vi "Shoot_object.vi"(7 "Shoot_states":T1, 8 "error in":errorcluster, 11 "DataIn":variant) -> (0 "error out":errorcluster)   [LabVIEW 2017]
uses:
  Shoot_states.ctl
  Shoot_data.ctl
  GameConfig/GameConfig_data.ctl
  ManageMovableObjects/HoldData/DataForColision.ctl
  ManageMovableObjects/HoldData/HoldData_mods.ctl
  Display/Display_mods.ctl
  ManageMovableObjects/ManRef_mods.ctl
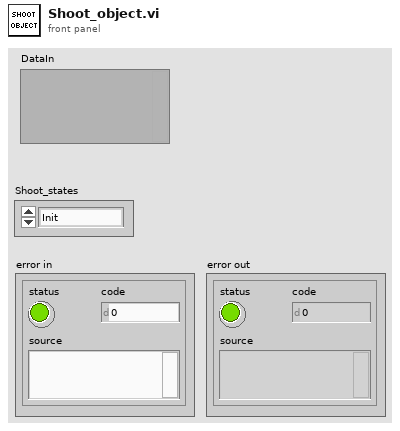
[diagram p1: front panel]
types:
  T1 = typedef "Shoot_states.ctl" = enum16{"Init", "Move", "Draw", "Destroy"}
  T2 = typedef "HoldData_mods.ctl" = enum16{"Init", "NewAster", "UpdateAster", "RemoveAster", "GetAsterData", "NewShoot", "UpdateShoot", "RemoveShoot", "GetShootData", "End"}
  T3 = typedef "DataForColision.ctl" = cluster{"X":dbl, "Y":dbl, "Size":dbl, "ID":i32}
  T4 = typedef "Shoot_data.ctl" = cluster{"Direction":dbl, "displayRef":refnum<vi>, "Max X":dbl, "Max Y":dbl, "Xpos":dbl, "Ypos":dbl, "ID":i32, "Config":T5}
  T5 = typedef "GameConfig_data.ctl" = cluster{"SpaceShip":cluster{"Angle":dbl, "SideLenght":dbl, "MaxLinearVeloc":dbl, "MaxAngularVeloc":dbl, "LinearAceleration":dbl, "AngularAceleration":dbl}, "Physics":cluster{"LinearDragFactor":dbl, "AngularDragFactor":dbl}, "Asteroids":cluster{"MaxSize":dbl, "MaxDivisions":i32, "MaxVeloc":dbl, "MinVeloc":dbl, "Fill":bool}, "Environment":cluster{"MaxAsteroids":i32, "TimeIncrement":dbl, "AsterProbCreation":dbl, "LogEnabled":bool}, "Shots":cluster{"MinTimeShots":dbl, "ShotSize":dbl, "ShotSpeed":dbl}}
  T6 = typedef "Display_mods.ctl" = enum16{"Init", "GetBase", "DrawAster", "DrawShip", "DrawShoot", "Clear", "Close"}
  T7 = cluster{"left":i16, "top":i16, "right":i16, "bottom":i16}
  T8 = typedef "ManRef_mods.ctl" = enum16{"Init", "NewAster", "MoveAll", "DestroyAster", "NewShoot", "DestroyShot", "CheckColision", "End"}
  T9 = typedef "LVBoundsTypeDef.ctl" = cluster{"Width":u32, "Height":u32}
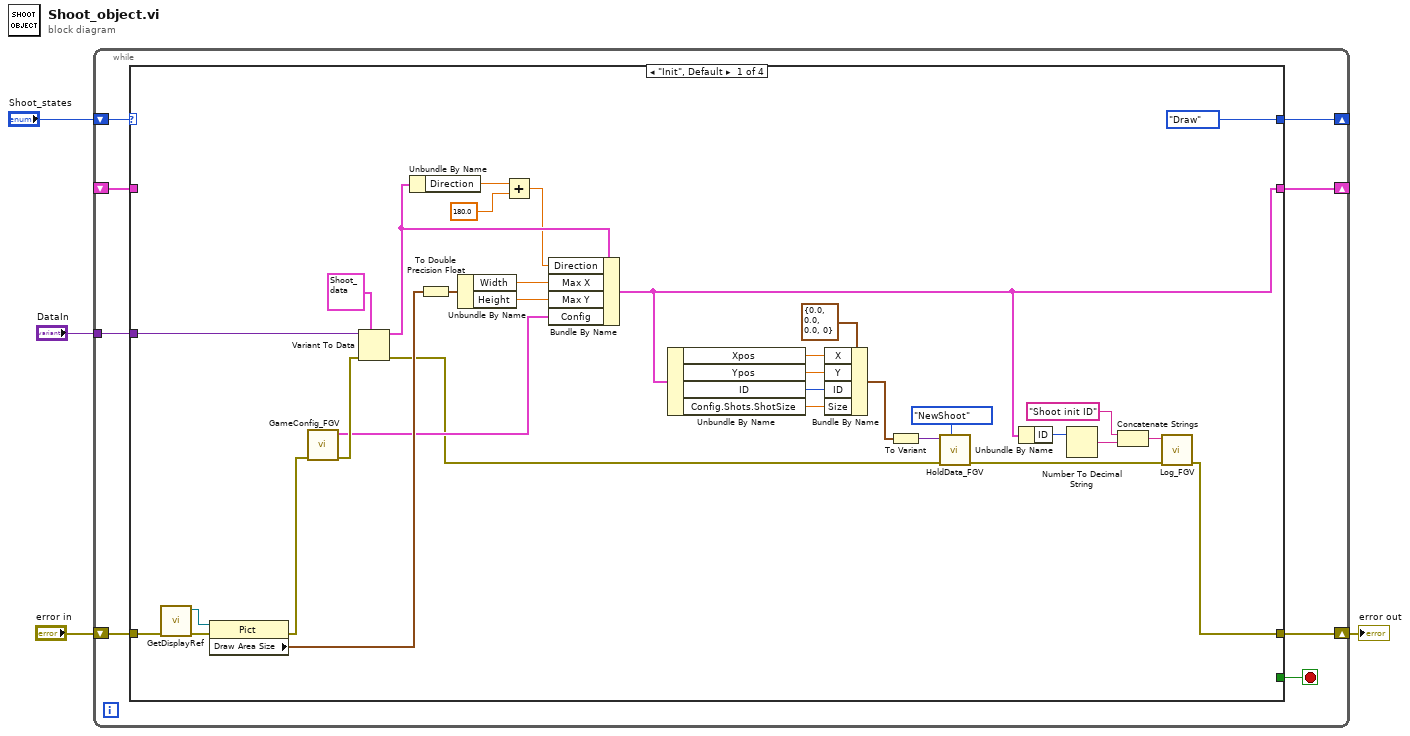
[diagram p0: block diagram]
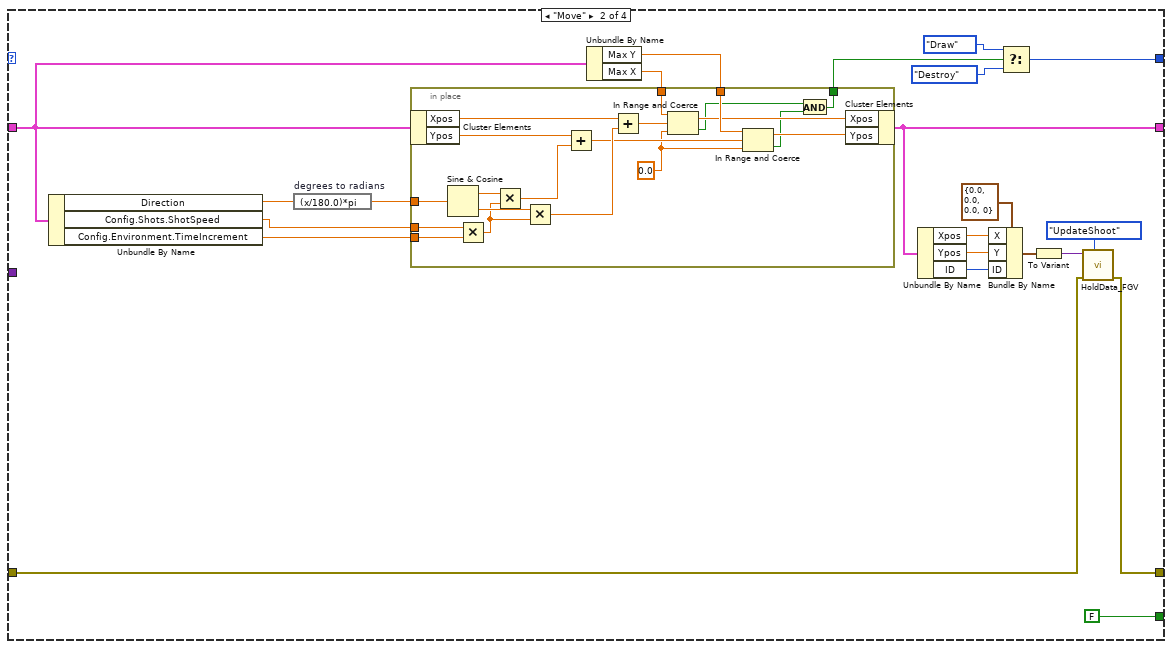
[diagram p2: hidden frame]
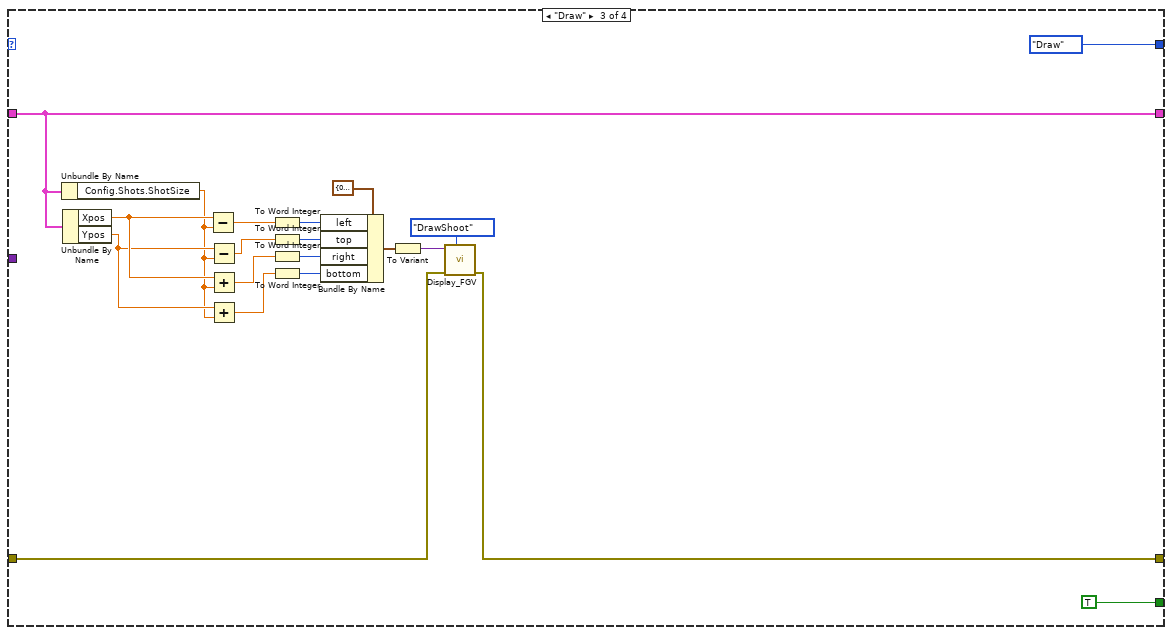
[diagram p3: hidden frame]
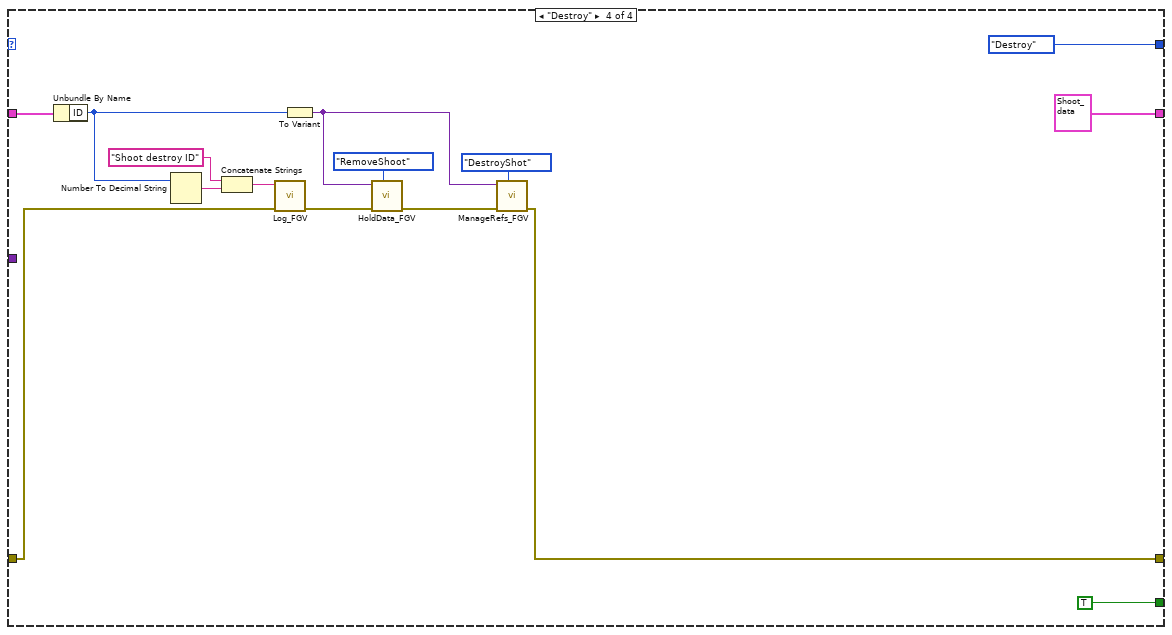
[diagram p4: hidden frame]
diagram:
  n1 = while {
    shift-right: [w10] -> w2
    shift-left: "error in" -> [w11]
    tunnel: "DataIn" -> [w9]
    shift-right: [w8] -> _
    shift-left: _ -> [w7]
    shift-right: [w6] -> _
    shift-left: "Shoot_states" -> [w12]
    stop <- w5 stop-if-true
    n2 = case shown="\"Init\", Default" w12 {
      tunnel: w11 -> [w45 w47 w92 w113]
      tunnel: [w28 w46 w95 w112] -> w10
      tunnel: w9 -> [w41 _ _ _]
      tunnel: [w16 w48 w94 T4 {"Direction"=0.0, "displayRef"=refnum, "Max X"=0.0, "Max Y"=0.0, "Xpos"=0.0, "Ypos"=0.0, "ID"=0, "Config"={"SpaceShip"={"Angle"=30.0, "SideLenght"=2.0, "MaxLinearVeloc"=10.0, "MaxAngularVeloc"=10.0, "LinearAceleration"=1.0, "AngularAceleration"=1.0}, "Physics"={"LinearDragFactor"=1.0, "AngularDragFactor"=1.0}, "Asteroids"={"MaxSize"=6.0, "MaxDivisions"=3, "MaxVeloc"=8.0, "MinVeloc"=1.0, "Fill"=FALSE}, "Environment"={"MaxAsteroids"=10, "TimeIncrement"=0.1, "AsterProbCreation"=0.1, "LogEnabled"=FALSE}, "Shots"={"MinTimeShots"=10.0, "ShotSize"=0.1, "ShotSpeed"=0.1}}} ("ShootData")] -> w8
      tunnel: w7 -> [_ w65 w94 w121]
      tunnel: [Shoot_states."Draw" ("Shoot_states 2") w58 Shoot_states."Draw" ("Shoot_states 2") Shoot_states."Destroy" ("Shoot_states 2")] -> w6
      tunnel: [_ FALSE TRUE TRUE] -> w5
      frame "Init", Default {
        n3 = call "GetDisplayRef.vi"("error in"=w45) -> ("error out"=w44:errorcluster, "Picture out"=w43:refnum<vi>)  [unwired: 9 in]
        n4 = property class="Pict"(reference=w43, error in=w44) -> (error out=w37:errorcluster, "Draw Area Size"=w42:T9)  [unwired: 1 out]
        n5 = call "GameConfig_FGV.vi"("error in"=w37) -> ("error out"=w36:errorcluster, "Config"=w35:T5)  [unwired: 9 in]
        n6 = Variant To Data(error in=w36, type=T4 {"Direction"=0.0, "displayRef"=refnum, "Max X"=0.0, "Max Y"=0.0, "Xpos"=0.0, "Ypos"=0.0, "ID"=0, "Config"={"SpaceShip"={"Angle"=30.0, "SideLenght"=2.0, "MaxLinearVeloc"=10.0, "MaxAngularVeloc"=10.0, "LinearAceleration"=1.0, "AngularAceleration"=1.0}, "Physics"={"LinearDragFactor"=1.0, "AngularDragFactor"=1.0}, "Asteroids"={"MaxSize"=6.0, "MaxDivisions"=3, "MaxVeloc"=8.0, "MinVeloc"=1.0, "Fill"=FALSE}, "Environment"={"MaxAsteroids"=10, "TimeIncrement"=0.1, "AsterProbCreation"=0.1, "LogEnabled"=FALSE}, "Shots"={"MinTimeShots"=10.0, "ShotSize"=0.1, "ShotSpeed"=0.1}}} ("ShootData"), Variant=w41) -> (data=w32:T4, error out=w14:errorcluster)
        n7 = Unbundle By Name(w32) -> ("Direction"=w31:dbl)
        n8 = To Double Precision Float(number=w42) -> (double precision float=w40:cluster{"Width":dbl, "Height":dbl})
        n9 = Unbundle By Name(w40) -> ("Width"=w39:dbl, "Height"=w38:dbl)
        n10 = Add(x=w31, y=180.0 ("x")) -> (x+y=w29:dbl)
        n11 = Bundle By Name(cluster=w32, "Direction"=w29, "Max X"=w39, "Max Y"=w38, "Config"=w35) -> (w16:T4)
        n12 = Unbundle By Name(w16) -> ("Xpos"=w22:dbl, "Ypos"=w21:dbl, "ID"=w20:i32, "Config.Shots.ShotSize"=w15:dbl)
        n13 = Bundle By Name(cluster=T3 {"X"=0.0, "Y"=0.0, "Size"=0.0, "ID"=0} ("DataForColision"), "X"=w22, "Y"=w21, "ID"=w20, "Size"=w15) -> (w19:T3)
        n14 = To Variant(anything=w19) -> (Variant=w18:variant)
        n15 = call "HoldData_FGV.vi"("HoldData_mods"=HoldData_mods."NewShoot", "error in"=w14, "DataIn"=w18) -> ("error out"=w13:errorcluster)  [unwired: 7 in, 1 out]
        n16 = Unbundle By Name(w16) -> ("ID"=w24:i32)
        n17 = Number To Decimal String(number=w24) -> (decimal integer string=w27:string)  [unwired: 1 in]
        n18 = Concatenate Strings("Shoot init ID" ("Log"), w27) -> (w25:string)
        n19 = call "Log_FGV.vi"("error in"=w13, "Log"=w25) -> ("error out"=w28:errorcluster)  [unwired: 9 in]
      }
      frame "Move" {
        n20 = Unbundle By Name(w65) -> ("Direction"=w57:dbl, "Config.Shots.ShotSpeed"=w67:dbl, "Config.Environment.TimeIncrement"=w66:dbl)
        n21 = expression code="(x/180.0)*pi" "degrees to radians"(w57) -> (w56:dbl)
        n22 = Unbundle By Name(w65) -> ("Max Y"=w63:dbl, "Max X"=w64:dbl)
        n23 = in-place {
          in-place-border: w67 -> [w87]
          in-place-border: w56 -> [w86]
          in-place-border: w66 -> [w78]
          in-place-border: w64 -> [w76]
          in-place-border: w63 -> [w74]
          in-place-border: [w68] -> w61
          w73 = 0.0 ("lower limit")
          n24 = in-place-cluster #1(w65) -> ("Xpos"=w79:dbl, "Ypos"=w82:dbl)
          n25 = Sine & Cosine(0:w86) -> (1:w83:dbl, 2:w85:dbl)
          n26 = Multiply(x=w87, y=w78) -> (x*y=w84:dbl)
          n27 = Multiply(x=w83, y=w84) -> (x*y=w81:dbl)
          n28 = Multiply(x=w85, y=w84) -> (x*y=w80:dbl)
          n29 = Add(x=w82, y=w81) -> (x+y=w75:dbl)
          n30 = Add(x=w79, y=w80) -> (x+y=w77:dbl)
          n31 = In Range and Coerce(upper limit=w76, x=w77, lower limit=w73) -> (coerced(x)=w71:dbl, In Range?=w69:bool)
          n32 = In Range and Coerce(upper limit=w74, x=w75, lower limit=w73) -> (coerced(x)=w72:dbl, In Range?=w70:bool)
          n33 = And(x=w69, y=w70) -> (x .and. y?=w68:bool)
          n34 = in-place-cluster #1("Xpos"=w71, "Ypos"=w72) -> (w48:T4)
        }
        n35 = Unbundle By Name(w48) -> ("Xpos"=w51:dbl, "Ypos"=w52:dbl, "ID"=w53:i32)
        n36 = Bundle By Name(cluster=T3 {"X"=0.0, "Y"=0.0, "Size"=0.0, "ID"=0} ("DataForColision"), "X"=w51, "Y"=w52, "ID"=w53) -> (w54:T3)
        n37 = Select(t=Shoot_states."Draw" ("Shoot_states 2"), s=w61, f=Shoot_states."Destroy" ("Shoot_states 2")) -> (s? t:f=w58:T1)
        n38 = To Variant(anything=w54) -> (Variant=w55:variant)
        n39 = call "HoldData_FGV.vi"("HoldData_mods"=HoldData_mods."UpdateShoot", "error in"=w47, "DataIn"=w55) -> ("error out"=w46:errorcluster)  [unwired: 7 in, 1 out]
      }
      frame "Draw" {
        n40 = Unbundle By Name(w94) -> ("Config.Shots.ShotSize"=w89:dbl)
        n41 = Unbundle By Name(w94) -> ("Xpos"=w102:dbl, "Ypos"=w101:dbl)
        n42 = Subtract(x=w102, y=w89) -> (x-y=w105:dbl)
        n43 = Subtract(x=w101, y=w89) -> (x-y=w103:dbl)
        n44 = Add(x=w102, y=w89) -> (x+y=w97:dbl)
        n45 = Add(x=w101, y=w89) -> (x+y=w96:dbl)
        n46 = To Word Integer(number=w105) -> (16bit integer=w104:i16)
        n47 = To Word Integer(number=w103) -> (16bit integer=w100:i16)
        n48 = To Word Integer(number=w97) -> (16bit integer=w99:i16)
        n49 = To Word Integer(number=w96) -> (16bit integer=w98:i16)
        n50 = Bundle By Name(cluster=T7 {"left"=0, "top"=0, "right"=0, "bottom"=0} ("rect"), "left"=w104, "top"=w100, "right"=w99, "bottom"=w98) -> (w88:T7)
        n51 = To Variant(anything=w88) -> (Variant=w91:variant)
        n52 = call "Display_FGV.vi"("Display_mods"=Display_mods."DrawShoot", "error in"=w92, "variant"=w91) -> ("error out"=w95:errorcluster)  [unwired: 7 in, 1 out]
      }
      frame "Destroy" {
        n53 = Unbundle By Name(w121) -> ("ID"=w114:i32)
        n54 = Number To Decimal String(number=w114) -> (decimal integer string=w117:string)  [unwired: 1 in]
        n55 = Concatenate Strings("Shoot destroy ID" ("Log"), w117) -> (w115:string)
        n56 = call "Log_FGV.vi"("error in"=w113, "Log"=w115) -> ("error out"=w109:errorcluster)  [unwired: 9 in]
        n57 = To Variant(anything=w114) -> (Variant=w110:variant)
        n58 = call "HoldData_FGV.vi"("HoldData_mods"=HoldData_mods."RemoveShoot", "error in"=w109, "DataIn"=w110) -> ("error out"=w108:errorcluster)  [unwired: 7 in, 1 out]
        n59 = call "ManageRefs_FGV.vi"("ManRef_mods"=ManRef_mods."DestroyShot", "error in"=w108, "DataIn"=w110) -> ("error out"=w112:errorcluster)  [unwired: 8 in]
      }
    }
  }
  "error out" <- w2
